vi "Main.vi"() -> ()   [LabVIEW 2018]
doc: "Simulates the DVD screensaver from all of our childhoods."
uses:
  <vilib>/picture/picture.llb/imagedata.ctl
  Controls/Cases.ctl
  Controls/DVD Data.ctl
  Controls/DVD Data items/Movement Direction - Horizontal.ctl
  Controls/DVD Data items/Movement Direction - Vertical.ctl
  Controls/DVD Data items/Movement Increment (pix).ctl
  Controls/DVD Data items/Time Delay (ms).ctl
  Controls/Logo Dimensions (pix).ctl
  Controls/Stage Dimensions (pix).ctl
  <vilib>/Utility/miscctls.llb/LVPointTypeDef.ctl
  <vilib>/Utility/miscctls.llb/LVBoundsTypeDef.ctl
panel:
  out "Cases":T1=enum."Moving"
  out "Image Data":T2
  out "Stage":picture
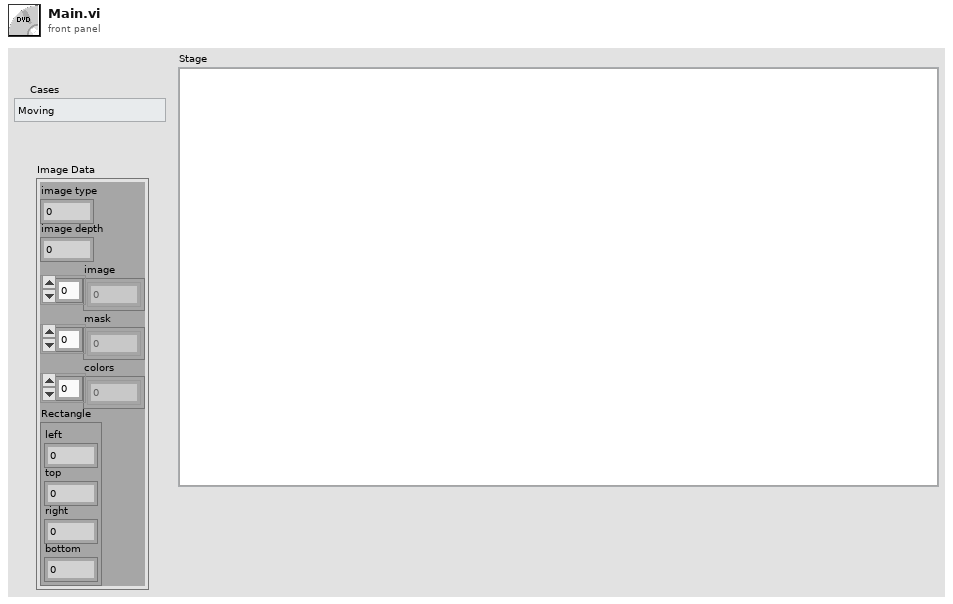
[diagram p1: front panel]
types:
  T1 = typedef "Cases.ctl" = enum16{"Initilisation", "Creating Stage", "Moving", "Checking if hit horizontally", "Checking if hit vertically", "Hitting top edge", "Hitting bottom edge", "Hitting left edge", "Hitting right edge"}
  T2 = typedef "imagedata.ctl" = cluster{"image type":i32, "image depth":i32, "image":u8[], "mask":u8[], "colors":u32[], "Rectangle":cluster{"left":i16, "top":i16, "right":i16, "bottom":i16}}
  T3 = typedef "DVD Data.ctl" = cluster{"Movement Data":cluster{"Movement Direction - Horizontal":T4, "Movement Direction - Vertical":T5, "Movement increment (pix)":T6, "Time delay (ms)":T7}, "Image Data":T2, "Logo Dimensions":T8, "Stage Dimensions":T9, "path to PNG file":path}
  T4 = typedef "Movement Direction - Horizontal.ctl" = enum16{"Left", "Right"}
  T5 = typedef "Movement Direction - Vertical.ctl" = enum16{"Up", "Down"}
  T6 = typedef "Movement Increment (pix).ctl" = i16
  T7 = typedef "Time Delay (ms).ctl" = u8
  T8 = typedef "Logo Dimensions (pix).ctl" = cluster{"X Dimension (pix)":i16, "Y Dimension (pix)":i16}
  T9 = typedef "Stage Dimensions (pix).ctl" = cluster{"X Dimension (pix)":i16, "Y Dimension (pix)":i16}
  T10 = typedef "LVPointTypeDef.ctl" = cluster{"Horizontal":i16, "Vertical":i16}
  T11 = typedef "LVBoundsTypeDef.ctl" = cluster{"Width":u32, "Height":u32}
  T12 = typedef "LVRectTypeDef.ctl" = cluster{"Left":i16, "Top":i16, "Right":i16, "Bottom":i16}
  T13 = cluster{"Movement Direction - Horizontal":T4, "Movement Direction - Vertical":T5, "Movement increment (pix)":T6, "Time delay (ms)":T7}
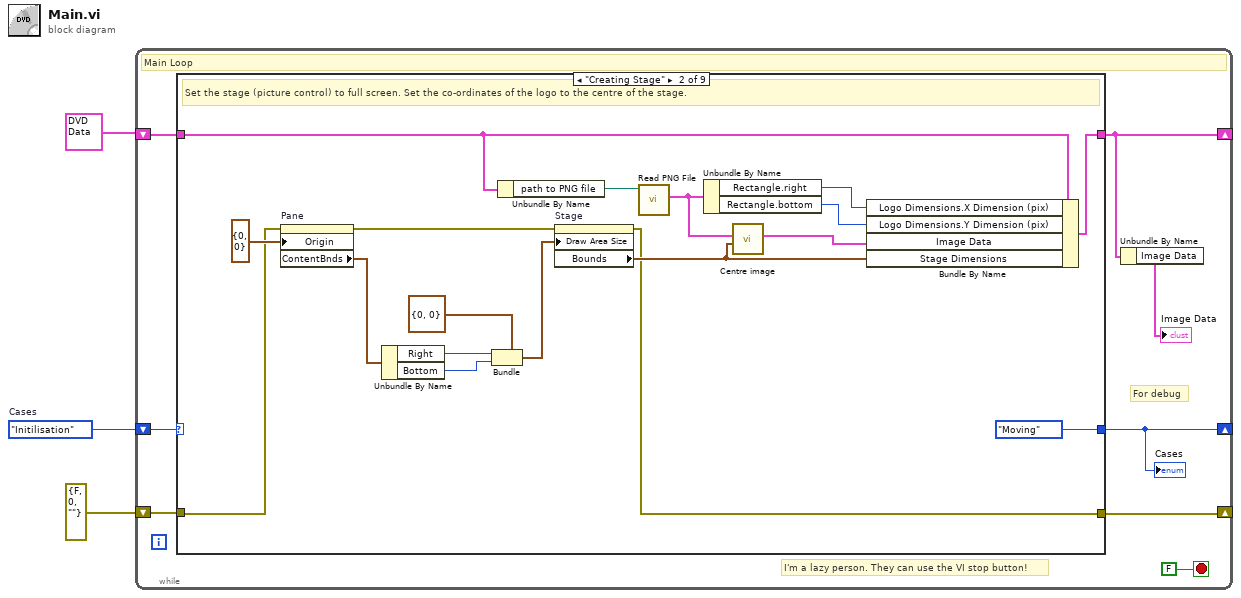
[diagram p0: block diagram]
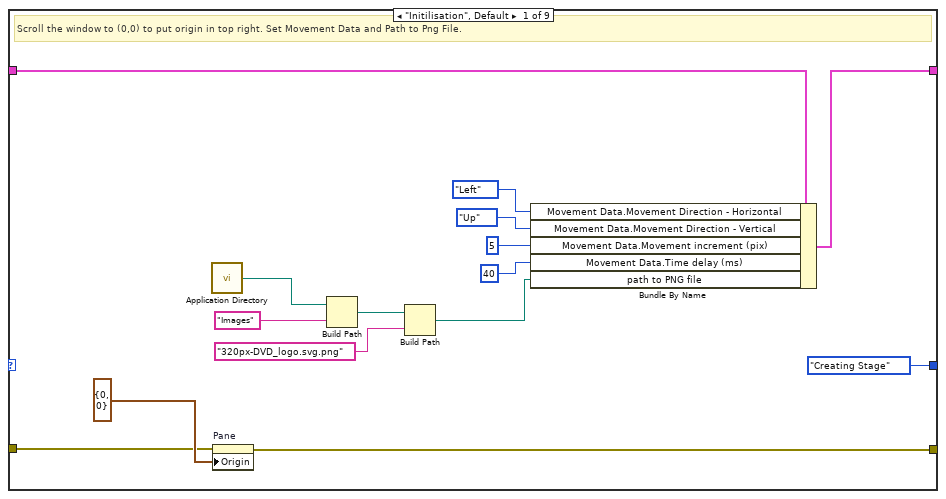
[diagram p2: hidden frame]
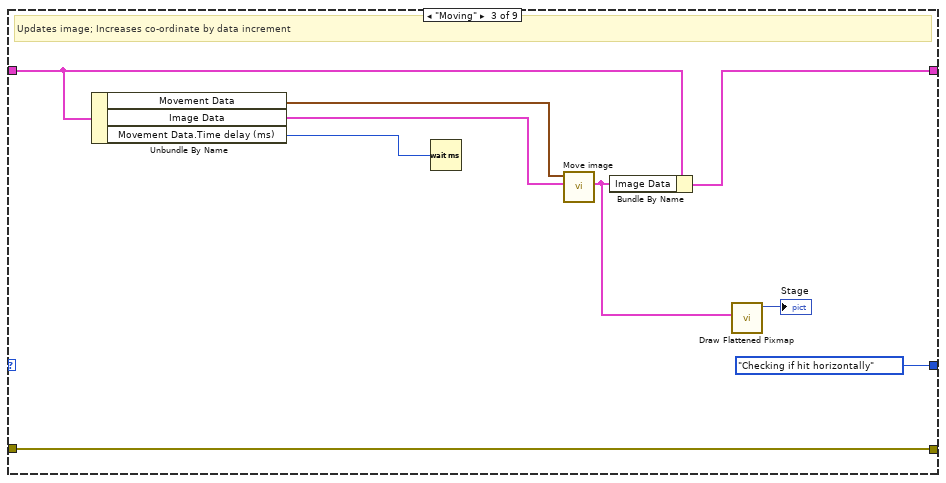
[diagram p3: hidden frame]
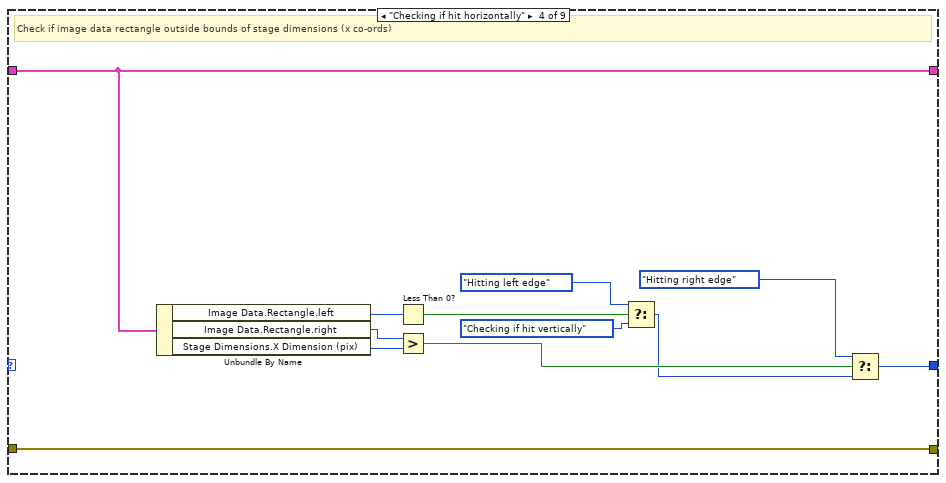
[diagram p4: hidden frame]
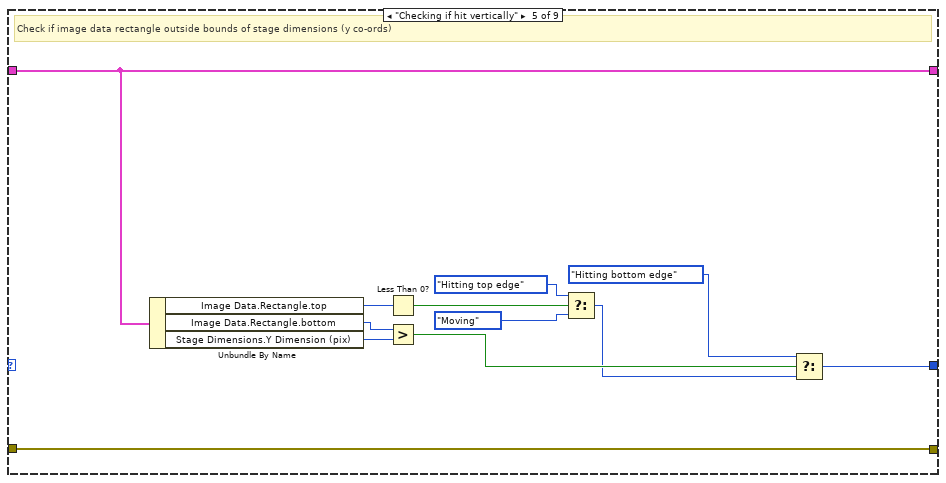
[diagram p5: hidden frame]
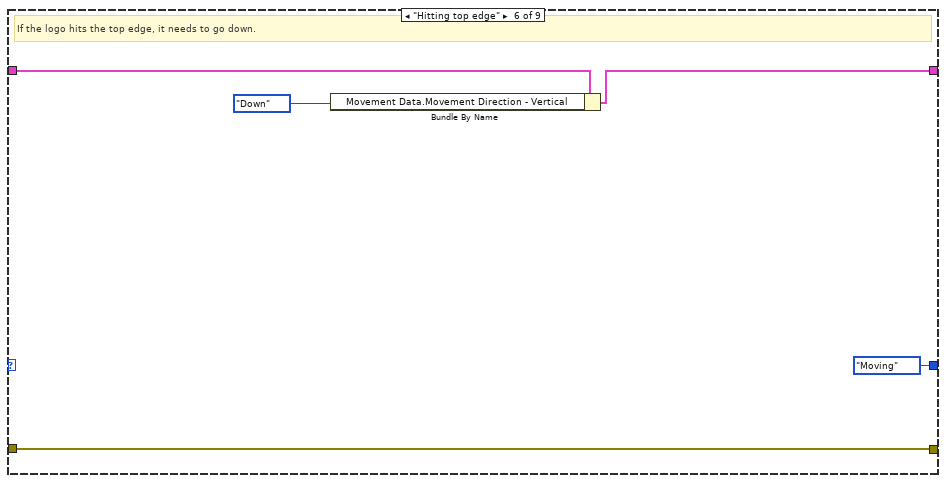
[diagram p6: hidden frame]
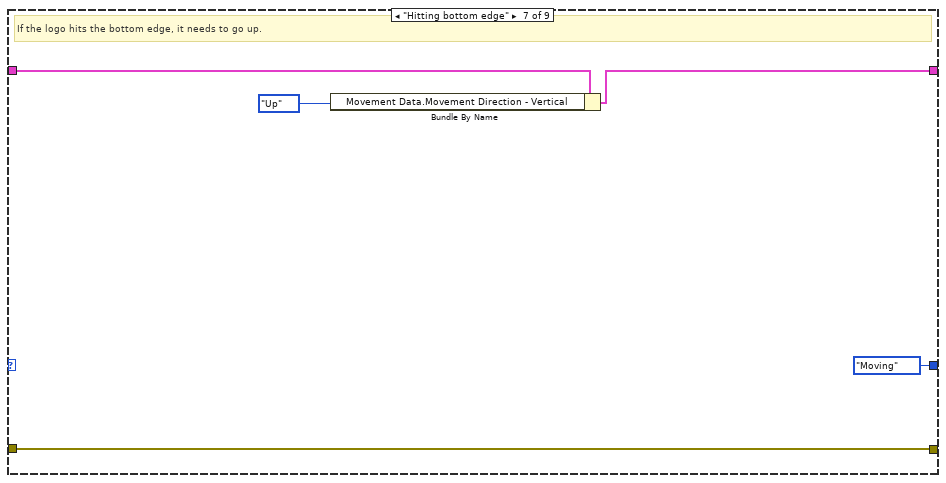
[diagram p7: hidden frame]
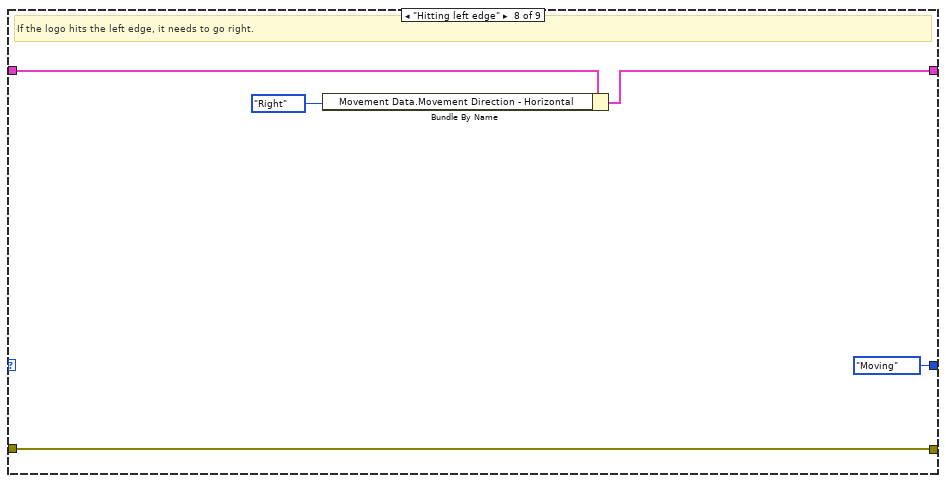
[diagram p8: hidden frame]
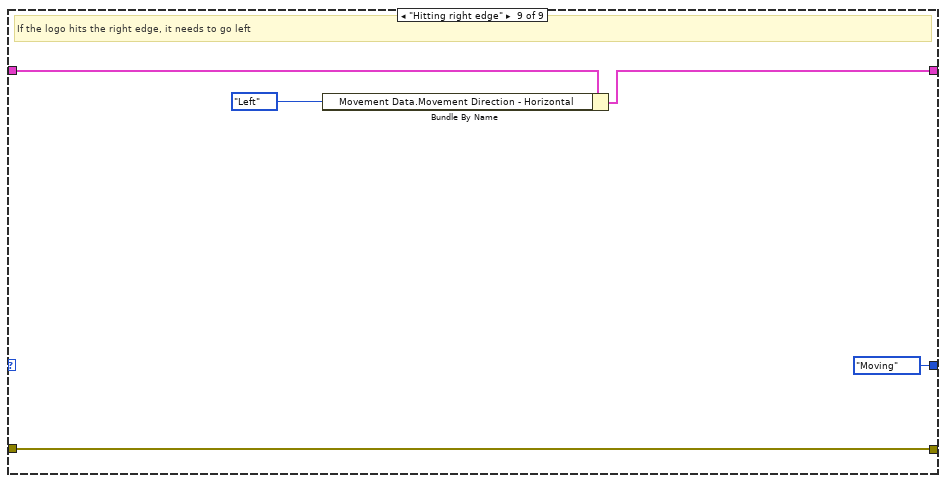
[diagram p9: hidden frame]
diagram:
  w3 = Cases."Initilisation"  # Cases
  n1 = while {
    shift-right: [w7] -> _
    shift-left: T3 {"Movement Data"={"Movement Direction - Horizontal"=enum."Left", "Movement Direction - Vertical"=enum."Up", "Movement increment (pix)"=0, "Time delay (ms)"=0}, "Image Data"={"image type"=0, "image depth"=0, "image"=[], "mask"=[], "colors"=[], "Rectangle"={"left"=0, "top"=0, "right"=0, "bottom"=0}}, "Logo Dimensions"={"X Dimension (pix)"=0, "Y Dimension (pix)"=0}, "Stage Dimensions"={"X Dimension (pix)"=0, "Y Dimension (pix)"=0}, "path to PNG file"=path ""} ("New data cluster") -> [w11]
    shift-right: [w10] -> _
    shift-left: errorcluster {"status"=FALSE, "code"=0, "source"=""} ("error out") -> [w9]
    shift-right: [w4] -> _
    shift-left: w3 -> [w5]
    stop <- FALSE stop-if-true
    # "For debug"
    # "I'm a lazy person. They can use the VI stop button!"
    # "Main Loop"
    n2 = case shown="\"Creating Stage\"" w5 {
      tunnel: [w26 w38 w50 w57 w69 w79 w84 w90 w95] -> w7
      tunnel: w11 -> [w20 w42 w51 w57 w69 w81 w86 w91 w96]
      tunnel: [w17 w28 w53 w65 w77 w82 w87 w92 w97] -> w10
      tunnel: w9 -> [w18 w27 w53 w65 w77 w82 w87 w92 w97]
      tunnel: [Cases."Creating Stage" ("Cases") Cases."Moving" ("Cases") Cases."Checking if hit horizontally" ("Cases") w54 w66 Cases."Moving" ("Cases") Cases."Moving" ("Cases") Cases."Moving" ("Cases") Cases."Moving" ("Cases")] -> w4
      frame "Initilisation", Default {
        # "Scroll the window to (0,0) to put origin in top right. Set Movement Data and Path to Png File."
        n3 = call <vilib>:"Application Directory.vi"() -> ("Application Directory"=w16:path)
        n4 = property on="Pane" class="Pane"(error in=w18, "Origin"=T10 {"Horizontal"=0, "Vertical"=0}) -> (error out=w17:errorcluster)  [unwired: 1 in, 1 out]
        n5 = Build Path(base path=w16, name or relative path="Images") -> (appended path=w14:path)
        n6 = Build Path(base path=w14, name or relative path="320px-DVD_logo.svg.png") -> (appended path=w12:path)
        n7 = Bundle By Name(cluster=w20, "Movement Data.Movement Direction - Horizontal"=Movement_Direction_-_Horizontal."Left" ("Movement Direction - Horizontal"), "Movement Data.Movement Direction - Vertical"=Movement_Direction_-_Vertical."Up" ("Movement Direction - Vertical"), "Movement Data.Movement increment (pix)"=T6 5 ("Movement increment (pix)"), "Movement Data.Time delay (ms)"=T7 40 ("Time delay (ms)"), "path to PNG file"=w12) -> (w26:T3)
      }
      frame "Creating Stage" {
        # "Set the stage (picture control) to full screen. Set the co-ordinates of the logo to the centre of the stage."
        n8 = property on="Pane" class="Pane"(error in=w27, "Origin"=T10 {"Horizontal"=0, "Vertical"=0}) -> (error out=w29:errorcluster, "ContentBnds"=w31:T12)  [unwired: 1 in, 1 out]
        n9 = Unbundle By Name(w31) -> ("Right"=w36:i16, "Bottom"=w35:i16)
        n10 = Bundle(cluster=T11 {"Width"=0, "Height"=0} ("Draw Area Size"), "Width"=w36, "Height"=w35) -> (w33:T11)
        n11 = Unbundle By Name(w42) -> ("path to PNG file"=w43:path)
        n12 = property on="Stage" class="Pict"(error in=w29, "Draw Area Size"=w33) -> (error out=w28:errorcluster, "Bounds"=w30:T11)  [unwired: 1 in, 1 out]
        n13 = call <vilib>:"Read PNG File.vi"("path to PNG file"=w43) -> ("image data"=w41:T2)  [unwired: 8 in, 2 out]
        n14 = Unbundle By Name(w41) -> ("Rectangle.right"=w40:i16, "Rectangle.bottom"=w39:i16)
        n15 = call "Centre image.vi"("Stage Dimensions"=w30, "Image data"=w41) -> ("Image Data"=w37:T2)  [unwired: 8 in]
        n16 = Bundle By Name(cluster=w42, "Logo Dimensions.X Dimension (pix)"=w40, "Logo Dimensions.Y Dimension (pix)"=w39, "Image Data"=w37, "Stage Dimensions"=w30) -> (w38:T3)
      }
      frame "Moving" {
        # "Updates image; Increases co-ordinate by data increment"
        n17 = Unbundle By Name(w51) -> ("Movement Data"=w46:T13, "Image Data"=w45:T2, "Movement Data.Time delay (ms)"=w48:T7)
        n18 = Wait (ms)(milliseconds to wait=w48) -> ()  [unwired: 1 out]
        n19 = call "Move image.vi"("Image Data"=w45, "Movement Data"=w46) -> ("Image Data"=w49:T2)  [unwired: 7 in]
        n20 = Bundle By Name(cluster=w51, "Image Data"=w49) -> (w50:T3)
        n21 = call <vilib>:"Draw Flattened Pixmap.vi"("image data"=w49) -> ("new picture"=→"Stage":picture)  [unwired: 8 in]
      }
      frame "Checking if hit horizontally" {
        # "Check if image data rectangle outside bounds of stage dimensions (x co-ords)"
        n22 = Unbundle By Name(w57) -> ("Image Data.Rectangle.left"=w64:i16, "Image Data.Rectangle.right"=w63:i16, "Stage Dimensions.X Dimension (pix)"=w62:i16)
        n23 = Less Than 0?(x=w64) -> (x < 0?=w59:bool)
        n24 = Greater?(x=w63, y=w62) -> (0:w58:bool)
        n25 = Select(t=Cases."Hitting left edge" ("Cases"), s=w59, f=Cases."Checking if hit vertically" ("Cases")) -> (s? t:f=w55:T1)
        n26 = Select(t=Cases."Hitting right edge" ("Cases"), s=w58, f=w55) -> (s? t:f=w54:T1)
      }
      frame "Checking if hit vertically" {
        # "Check if image data rectangle outside bounds of stage dimensions (y co-ords)"
        n27 = Unbundle By Name(w69) -> ("Image Data.Rectangle.top"=w76:i16, "Image Data.Rectangle.bottom"=w75:i16, "Stage Dimensions.Y Dimension (pix)"=w74:i16)
        n28 = Less Than 0?(x=w76) -> (x < 0?=w71:bool)
        n29 = Greater?(x=w75, y=w74) -> (0:w70:bool)
        n30 = Select(t=Cases."Hitting top edge" ("Cases"), s=w71, f=Cases."Moving" ("Cases")) -> (s? t:f=w67:T1)
        n31 = Select(t=Cases."Hitting bottom edge" ("Cases"), s=w70, f=w67) -> (s? t:f=w66:T1)
      }
      frame "Hitting top edge" {
        # "If the logo hits the top edge, it needs to go down."
        n32 = Bundle By Name(cluster=w81, "Movement Data.Movement Direction - Vertical"=Movement_Direction_-_Vertical."Down" ("Movement Direction - Vertical")) -> (w79:T3)
      }
      frame "Hitting bottom edge" {
        # "If the logo hits the bottom edge, it needs to go up."
        n33 = Bundle By Name(cluster=w86, "Movement Data.Movement Direction - Vertical"=Movement_Direction_-_Vertical."Up" ("Movement Direction - Vertical")) -> (w84:T3)
      }
      frame "Hitting left edge" {
        # "If the logo hits the left edge, it needs to go right."
        n34 = Bundle By Name(cluster=w91, "Movement Data.Movement Direction - Horizontal"=Movement_Direction_-_Horizontal."Right" ("Movement Direction - Horizontal")) -> (w90:T3)
      }
      frame "Hitting right edge" {
        # "If the logo hits the right edge, it needs to go left"
        n35 = Bundle By Name(cluster=w96, "Movement Data.Movement Direction - Horizontal"=Movement_Direction_-_Horizontal."Left" ("Movement Direction - Horizontal")) -> (w95:T3)
      }
    }
    "Cases" <- w4
    n36 = Unbundle By Name(w7) -> ("Image Data"=→"Image Data":T2)
  }
